vi "GetSerialIncoming.vi"(8 "error in (no error)":errorcluster, 10 "Input buffer refnum":refnum<vi>, 11 "VISAResourceName in":refnum<vi>) -> (0 "error out":errorcluster)   [LabVIEW 2016]
panel:
  # "Looks for incoming data on a serial port specified by the VISA refnum.\nIf an error would occur, a Stop-command is appended to the command \nqueue. To stop it, send TRUE to the Stop-notifier.\n\nMagne Lauritzen 2016"
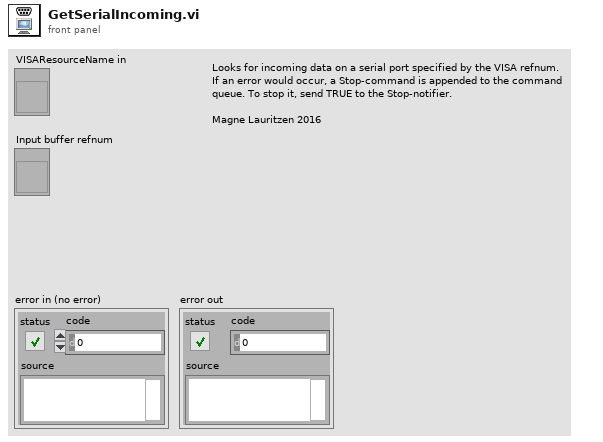
[diagram p1: front panel]
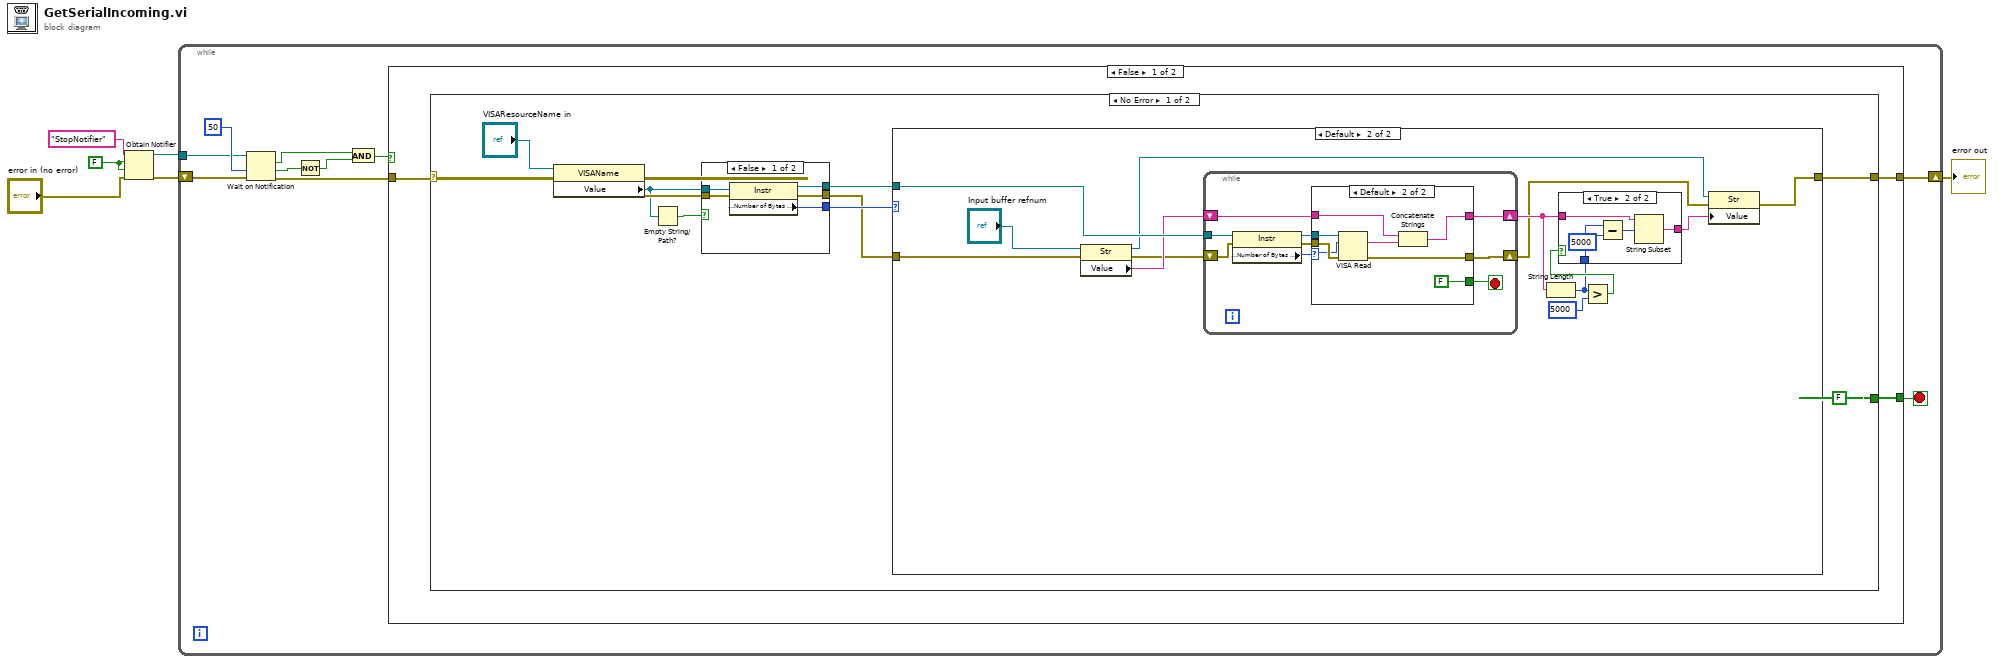
[diagram p0: block diagram]
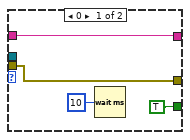
[diagram p4: hidden frame]
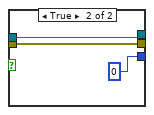
[diagram p5: hidden frame]
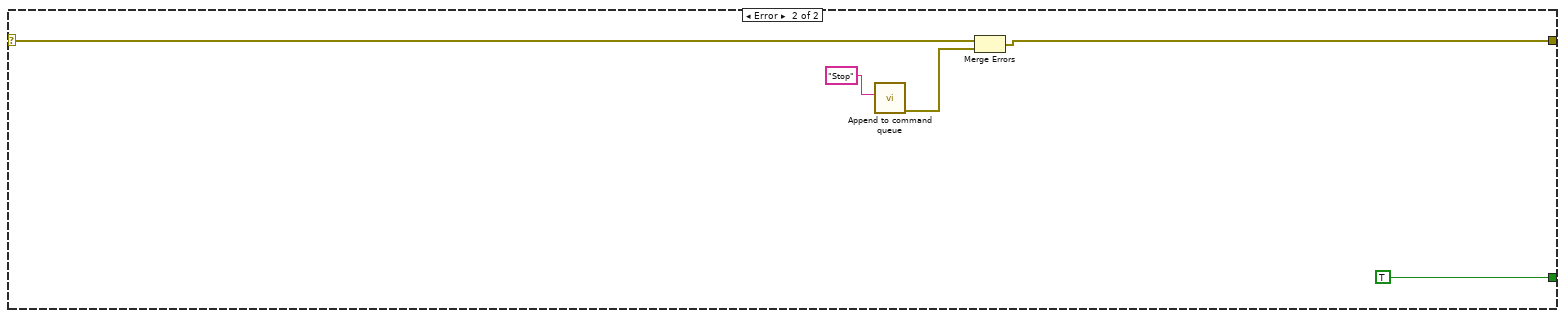
[diagram p6: hidden frame]
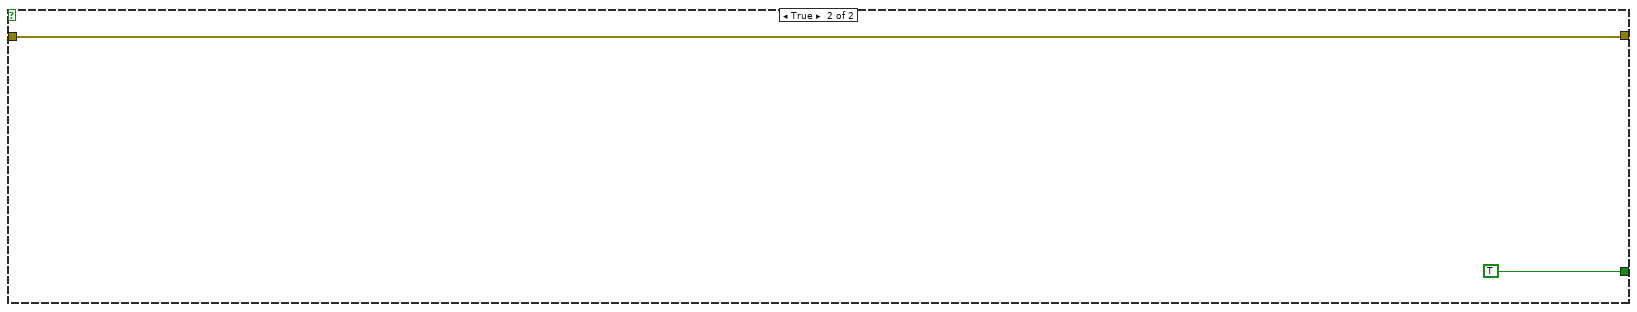
[diagram p7: hidden frame]
diagram:
  w5 = FALSE
  n1 = Obtain Notifier(name (unnamed)="StopNotifier", notification data type=w5, create if not found? (T)=w5, error in (no error)="error in (no error)") -> (notifier out=w3:refnum<notifier>, error out=w2:errorcluster)  [unwired: 1 out]
  n2 = while {
    shift-right: [w16] -> w6
    shift-left: w2 -> [w14]
    tunnel: w3 -> [w7]
    stop <- w8 stop-if-true
    n3 = Wait on Notification(notifier=w7, timeout in ms (-1)=u32 50 ("milliseconds to wait"), error in (no error)=w14) -> (notification=w11:bool, timed out?=w13:bool, error out=w9:errorcluster)  [unwired: 1 in, 1 out]
    n4 = Not(x=w13) -> (.not. x?=w12:bool)
    n5 = And(x=w11, y=w12) -> (x .and. y?=w10:bool)
    n6 = case shown="False" w10 {
      tunnel: [w19 w84] -> w16
      tunnel: w9 -> [w18 w84]
      tunnel: [w17 TRUE] -> w8
      frame False {
        n7 = case shown="No Error" w18 {
          selector: w18 -> [w24 w82]
          tunnel: [w25 w81] -> w19
          tunnel: [FALSE TRUE] -> w17
          frame No Error {
            n8 = property on="Property Node" class="VISAName"(reference="VISAResourceName in", error in=w24) -> (error out=w29:errorcluster, "Value"=w22:refnum<visa-resource-name>)  [unwired: 1 out]
            n9 = Empty String/Path?(string/path=w22) -> (empty?=w21:bool)
            n10 = case shown="False" w21 {
              tunnel: w29 -> [w75 w77]
              tunnel: [w74 u32 0 ("Bytes at Port")] -> w28
              tunnel: [w73 w76] -> w27
              tunnel: [w72 w77] -> w26
              tunnel: w22 -> [w71 w76]
              frame False {
                n11 = property class="Instr"(reference=w71, error in=w75) -> (reference out=w73:refnum<visa-resource-name>, error out=w72:errorcluster, "Serial Settings:Number of Bytes at Serial Port"=w74:u32)
              }
              frame True {
              }
            }
            n12 = case shown="Default" w28 {
              tunnel: w27 -> [_ w43]
              tunnel: w26 -> [w30 w39]
              tunnel: [w30 w42] -> w25
              frame 0 {
              }
              frame Default {
                n13 = property on="Property Node" class="Str"(reference="Input buffer refnum", error in=w39) -> (reference out=w37:refnum<vi>, error out=w40:errorcluster, "Value"=w41:string)
                n14 = while {
                  shift-right: [w55] -> w33
                  shift-left: w41 -> [w56]
                  shift-right: [w52] -> w31
                  shift-left: w40 -> [w51]
                  tunnel: w43 -> [w50]
                  stop <- w57 stop-if-true
                  n15 = property class="Instr"(reference=w50, error in=w51) -> (reference out=w54:refnum<visa-resource-name>, error out=w53:errorcluster, "Serial Settings:Number of Bytes at Serial Port"=w58:u32)
                  n16 = case shown="Default" w58 {
                    selector: w58 -> [_ w64]
                    tunnel: [TRUE FALSE] -> w57
                    tunnel: w56 -> [w61 w68]
                    tunnel: [w61 w69] -> w55
                    tunnel: w54 -> [_ w70]
                    tunnel: w53 -> [w60 w65]
                    tunnel: [w60 w63] -> w52
                    frame 0 {
                      n17 = Wait (ms)(milliseconds to wait=u32 10) -> ()  [unwired: 1 out]
                    }
                    frame Default {
                      n18 = VISA Read(VISA resource name=w70, byte count=w64, error in (no error)=w65) -> (read buffer=w67:string, error out=w63:errorcluster)  [unwired: 2 out]
                      n19 = Concatenate Strings(w68, w67) -> (w69:string)
                    }
                  }
                }
                n20 = String Length(string=w33) -> (length=w34:i32)
                n21 = Greater?(x=w34, y=5000) -> (0:w35:bool)
                n22 = case shown="True" w35 {
                  tunnel: w34 -> [_ w49]
                  tunnel: w33 -> [w44 w46]
                  tunnel: [w44 w45] -> w32
                  frame False {
                  }
                  frame True {
                    n23 = Subtract(x=w49, y=5000) -> (x-y=w47:i32)
                    n24 = String Subset(string=w46, offset (0)=w47) -> (substring=w45:string)  [unwired: 1 in]
                  }
                }
                n25 = property on="Property Node" class="Str"(reference=w37, error in=w31, "Value"=w32) -> (error out=w42:errorcluster)  [unwired: 1 out]
              }
            }
          }
          frame Error {
            n26 = call "Append to command queue.vi"("Single command"="Stop") -> ("error out"=w80:errorcluster)  [unwired: 10 in]
            n27 = Merge Errors(w82, w80) -> (w81:errorcluster)
          }
        }
      }
      frame True {
      }
    }
  }
  "error out" <- w6
